vi "Set Motor Speed.vi"(6 "Ramp Time":dbl[unit], 7 "Mono System # (0)":T1, 8 "error in (no error)":errorcluster, 9 "Max Frequency":dbl[unit], 10 "Min Frequency":dbl[unit], 11 "VISA resource name":refnum<visa-resource-name>) -> ()   [LabVIEW 2009, in "JY-SPEX-TRIAX.lvlib"]
doc: "Sets the minimum and maximum motor speeds and the time to ramp from the min to the max."
uses:
  JY-SPEX-TRIAX.lvlib
  controls.llb/Monochromator System Number.ctl
panel:
  out "error out":errorcluster
  out "VISA resource name out":refnum<visa-resource-name>
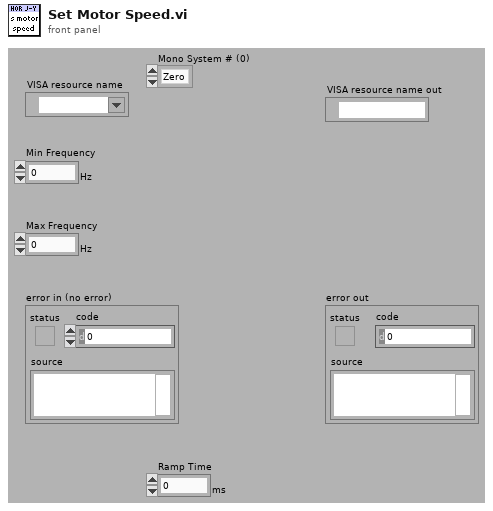
[diagram p1: front panel]
types:
  T1 = typedef "JY-SPEX-TRIAX.lvlib/Monochromator System Number.ctl" = enum16{"Zero", "One"}
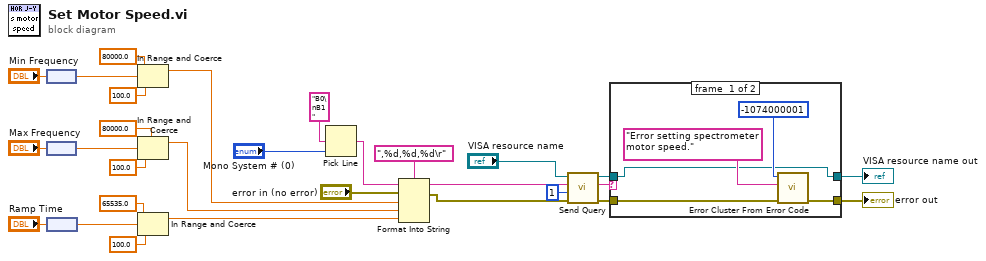
[diagram p0: block diagram]
diagram:
  n1 = node("Min Frequency") -> (w26:dbl)
  n2 = node("Max Frequency") -> (w23:dbl)
  n3 = node("Ramp Time") -> (w20:dbl)
  n4 = In Range and Coerce(upper limit=80000.0, x=w26, lower limit=100.0) -> (coerced(x)=w13:dbl)  [unwired: 1 out]
  n5 = In Range and Coerce(upper limit=80000.0, x=w23, lower limit=100.0) -> (coerced(x)=w12:dbl)  [unwired: 1 out]
  n6 = In Range and Coerce(upper limit=65535.0, x=w20, lower limit=100.0) -> (coerced(x)=w11:dbl)  [unwired: 1 out]
  n7 = Pick Line(multi-line string="B0\nB1", line index="Mono System # (0)") -> (output string=w15:string)  [unwired: 1 out]
  n8 = Format Into String(format string=",%d,%d,%d\r", initial string=w15, error in="error in (no error)", w13, w12, w11) -> (resulting string=w10:string, error out=w7:errorcluster)
  n9 = call "Send Query.vi"("error in (no error)"=w7, "byte count"=u32 1, "write buffer"=w10, "VISA resource name"="VISA resource name") -> ("error out"=w2:errorcluster, "read buffer"=w5:string, "VISA resource name out"=w4:refnum<visa-resource-name>)  [unwired: 5 out]
  n10 = case shown="Default" w5 {
    tunnel: w4 -> [w30 w36]
    tunnel: [w30 w36] -> w3
    tunnel: w2 -> [w32 w35]
    tunnel: [w31 w35] -> w1
    frame #0 {
      n11 = call <vilib>:"Error Cluster From Error Code.vi"("error in (no error)"=w32, "error message (\"\")"="Error setting spectrometer motor speed." ("error message (\"\")"), "error code (0)"=-1074000001) -> ("error out"=w31:errorcluster)  [unwired: 1 in, 5 out]
    }
    frame #1 {
    }
  }
  "VISA resource name out" <- w3
  "error out" <- w1
